vi "save_xml.vi"(8 "error in":errorcluster, 10 "base path":path, 11 "Analog Output Parameters":T1={"Enable Analog Out?"=TRUE, "Physical Channel"="PXI1Slot2/ao0:2", "Minimum Value"=-10.0, "Maximum Value"=10.0, "Samples per second"=10000.0, "Total AO Time (seconds)"="p", "Analog Output Equations for each Channel"=[], "Start Trigger"={"Wait for start trigger?"=FALSE, "source"="/Dev1/PFI0", "edge"=10280}} {"Start Trigger"."edge" items=["Rising"=10280, "Falling"=10171]; "Maximum Value" format="%0.2f"; "Minimum Value" format="%0.2f"}) -> (0 "error out":errorcluster)   [LabVIEW 2012, in "Analog_Output.lvclass"]
uses:
  Analog_Output.lvclass
  AO_settings.ctl
  <vilib>/Utility/xml.llb/Write to XML File(string).vi
panel:
  # "You may use formulas here.  If 't' is not specified in the variable or parameter tables, it will be used here as time in seconds.\nIn addition to the usual functions (sin(), cos(), etc.) you may also use spike(), square() and step(), \nNote, analog output will continue until Total AO Time runs out, or Measurement Timeout is reached, \neven if HSDIO pulses or DAQmx pulses have finished."
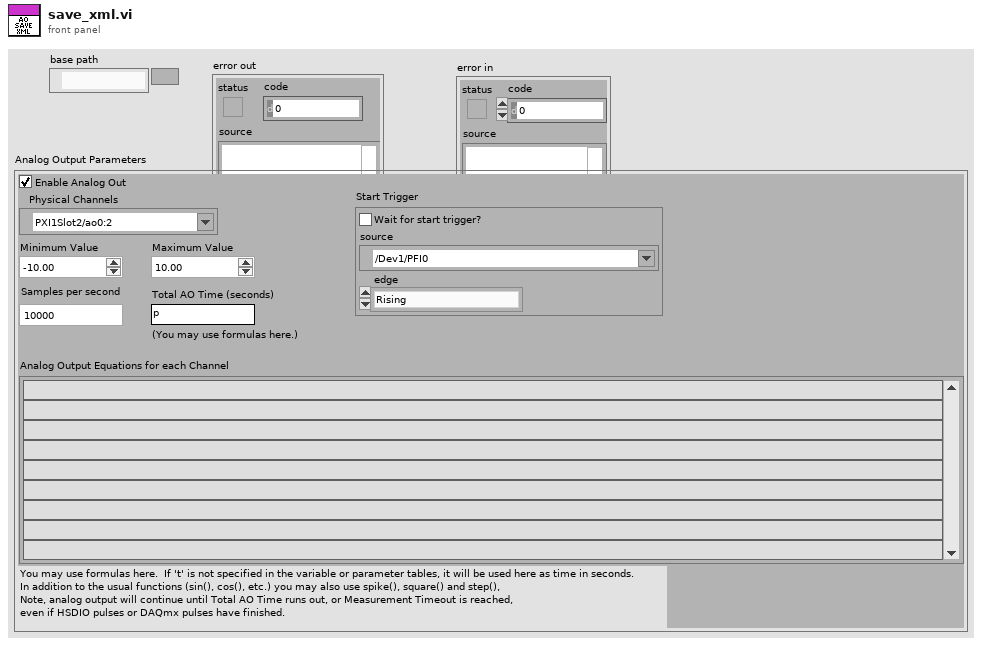
[diagram p1: front panel]
types:
  T1 = typedef "Analog_Output.lvclass/AO_settings.ctl" = cluster{"Enable Analog Out?":bool, "Physical Channel":tag, "Minimum Value":dbl, "Maximum Value":dbl, "Samples per second":dbl, "Total AO Time (seconds)":string, "Analog Output Equations for each Channel":string[], "Start Trigger":cluster{"Wait for start trigger?":bool, "source":tag, "edge":i32}}
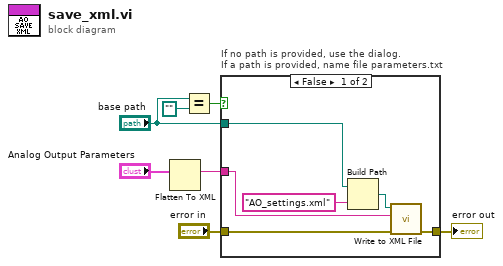
[diagram p0: block diagram]
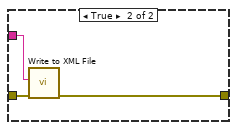
[diagram p2: hidden frame]
diagram:
  n1 = Flatten To XML(anything="Analog Output Parameters") -> (xml string=w2:string)
  n2 = Equal?(x="base path", y=path "") -> (x = y?=w5:bool)
  n3 = case "If no path is provided, use the dialog.\nIf a path is provided, name file parameters.txt" shown="False" w5 {
    tunnel: [w9 w15] -> w6
    tunnel: "base path" -> [w12 _]
    tunnel: "error in" -> [w10 w16]
    tunnel: w2 -> [w8 w14]
    frame False {
      n4 = Build Path(base path=w12, name or relative path="AO_settings.xml") -> (appended path=w11:path)
      n5 = call-poly <vilib>:"Write to XML File.vi"("error in (no error)"=w10, "XML Input"=w8, "XML File Path"=w11) -> ("error out"=w9:errorcluster)  [unwired: 6 in, 2 out]
    }
    frame True {
      n6 = call-poly <vilib>:"Write to XML File.vi"("error in (no error)"=w16, "XML Input"=w14) -> ("error out"=w15:errorcluster)  [unwired: 7 in, 2 out]
    }
  }
  "error out" <- w6
